vi "Analyze GB.vi"(8 "Integer Tolerance":dbl=0.1, 9 "Twist Angle (Deg)":dbl=60.0, 10 "Grain 2 Orientation":dbl[](array[numeric])=[1.0, 1.0, 1.0], 11 "Grain 1 Orientation":dbl[](array[numeric])=[1.0, 1.0, 1.0]) -> (0 "Misorientation Angle":dbl, 1 "Misorientation Axis, o":dbl[](array[numeric])=[1.0, 1.0, 1.0], 2 "Grain 2 Integers":dbl[](array[numeric])=[1.0, 1.0, 1.0], 3 "Grain 1 Integers":dbl[](array[numeric])=[1.0, 1.0, 1.0], 4 "Tilt Angle (Deg)":dbl, 5 "Suggested Viewing Angle":dbl[](array[numeric])=[1.0, 1.0, 1.0], 6 "Misorientation Matrix":T1, 7 "Viewable?":bool)   [LabVIEW 2010]
uses:
  <vilib>/Analysis/Matrix/Datatypes/RealMatrix.ctl
  <vilib>/Analysis/baseanly.llb/Real A x B.vi
  <vilib>/Analysis/_algsub.llb/Real Matrix Trace.vi
  <vilib>/Analysis/NI_AALPro.lvlib
  <vilib>/Analysis/NI_AALBase.lvlib
  <vilib>/Analysis/Matrix/NI_Matrix.lvlib
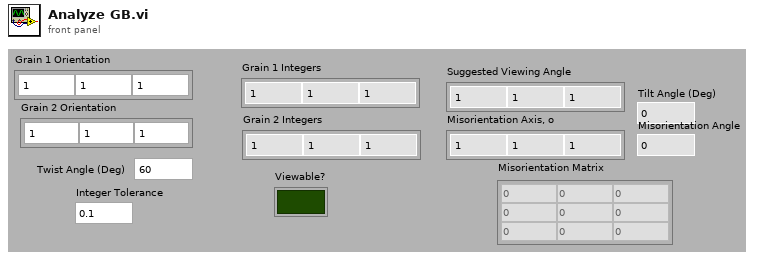
[diagram p1: front panel]
types:
  T1 = typedef "NI_Matrix.lvlib/RealMatrix.ctl" = dbl[][]
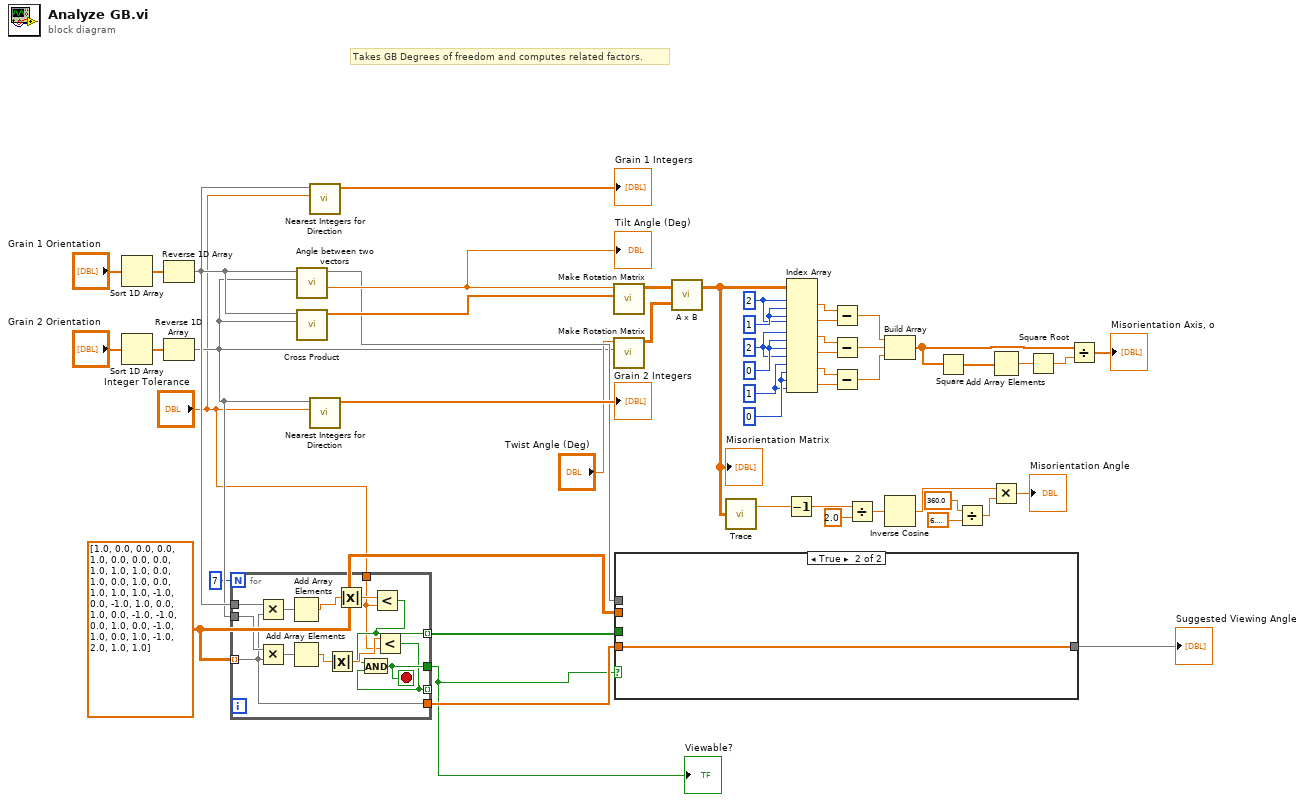
[diagram p0: block diagram]
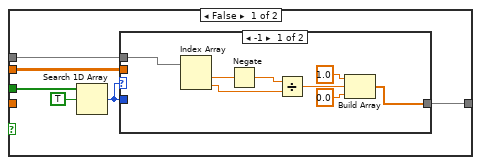
[diagram p2: hidden frame]
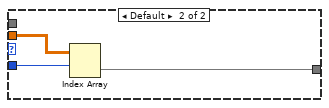
[diagram p3: hidden frame]
diagram:
  w21 = 0 ("index (row)")
  w20 = 1 ("index (row)")
  w23 = 0 ("disabled index (col)")
  w22 = 2 ("index (row)")
  w25 = 1 ("disabled index (col)")
  w24 = 2 ("index (row)")
  w45 = dbl[][] [[1.0, 0.0, 0.0], [0.0, 1.0, 0.0], [0.0, 0.0, 1.0], [1.0, 1.0, 0.0], [1.0, 0.0, 1.0], [0.0, 1.0, 1.0], [1.0, -1.0, 0.0], [-1.0, 1.0, 0.0], [1.0, 0.0, -1.0], [-1.0, 0.0, 1.0], [0.0, -1.0, 1.0], [0.0, 1.0, -1.0], [2.0, 1.0, 1.0]] ("Grain 1 Orientation 2")
  # "Takes GB Degrees of freedom and computes related factors."
  n1 = Sort 1D Array(array="Grain 1 Orientation") -> (sorted array=w48:dbl[])
  n2 = Sort 1D Array(array="Grain 2 Orientation") -> (sorted array=w47:dbl[])
  n3 = Reverse 1D Array(array=w48) -> (reversed array=w13:dbl[])
  n4 = Reverse 1D Array(array=w47) -> (reversed array=w4:dbl[])
  n5 = for {
    N: 7 -> [_]
    tunnel: w13 -> [w62]
    tunnel: w45 -> [w58] mode=indexing
    tunnel: [w58] -> w43
    tunnel: w4 -> [w59]
    tunnel: [w53] -> w46 mode=indexing
    tunnel: [w52] -> _ mode=indexing
    tunnel: [w63] -> w3
    tunnel: "Integer Tolerance" -> [w51]
    stop <- w63 stop-if-true
    n6 = Multiply(x=w62, y=w58) -> (x*y=w61:dbl[])
    n7 = Multiply(x=w59, y=w58) -> (x*y=w60:dbl[])
    n8 = Add Array Elements(numeric array=w61) -> (sum=w57:dbl)
    n9 = Add Array Elements(numeric array=w60) -> (sum=w56:dbl)
    n10 = Absolute Value(x=w56) -> (abs(x)=w54:dbl)
    n11 = Absolute Value(x=w57) -> (abs(x)=w55:dbl)
    n12 = Less?(x=w55, y=w51) -> (x < y?=w53:bool)
    n13 = Less?(x=w54, y=w51) -> (x < y?=w52:bool)
    n14 = And(x=w53, y=w52) -> (x .and. y?=w63:bool)
  }
  "Viewable?" <- w3
  n15 = call "Angle between two vectors.vi"("Vector 2"=w4, "Vector 1"=w13) -> ("Angle (Degrees)"=w30:dbl)  [unwired: 7 in, 2 out]
  "Tilt Angle (Deg)" <- w30
  n16 = call <vilib>:"Cross Product.vi"("B Vector"=w4, "A Vector"=w13) -> ("Cross Product"=w31:dbl[])  [unwired: 8 in, 1 out]
  n17 = call "Nearest Integers for Direction.vi"("Tolerance"="Integer Tolerance", "Direction"=w13) -> ("Nearest Integer Directions"=→"Grain 1 Integers":dbl[])  [unwired: 8 in, 1 out]
  n18 = call "Nearest Integers for Direction.vi"("Tolerance"="Integer Tolerance", "Direction"=w4) -> ("Nearest Integer Directions"=→"Grain 2 Integers":dbl[])  [unwired: 8 in, 1 out]
  n19 = call "Make Rotation Matrix.vi"("Rotation Axis"=w31, "Rotation Angle (Degree)"=w30) -> ("Rotation Matrix"=w32:T1)  [unwired: 9 in]
  n20 = call "Make Rotation Matrix.vi"("Rotation Axis"=w4, "Rotation Angle (Degree)"="Twist Angle (Deg)") -> ("Rotation Matrix"=w42:T1)  [unwired: 9 in]
  n21 = case shown="True" w3 {
    tunnel: [w66 w81] -> w44
    tunnel: w46 -> [w69 _]
    tunnel: w45 -> [w67 _]
    tunnel: w13 -> [w64 _]
    tunnel: w43 -> [_ w81]
    frame False {
      n22 = Search 1D Array(1D array=w69, element=TRUE) -> (index of element=w65:i32)  [unwired: 1 in]
      n23 = case shown="-1" w65 {
        tunnel: w67 -> [_ w80]
        tunnel: w65 -> [_ w79]
        tunnel: [w74 w78] -> w66
        tunnel: w64 -> [w77 _]
        frame -1 {
          n24 = Index Array(array=w77) -> (element #1=w72:dbl, element #2=w73:dbl)  [unwired: 2 in]
          n25 = Negate(x=w72) -> (-x=w71:dbl)
          n26 = Divide(x=w71, y=w73) -> (x/y=w70:dbl)
          n27 = Build Array(1.0 ("element"), w70, 0.0 ("element")) -> (w74:dbl[])
        }
        frame Default {
          n28 = Index Array(array=w80, index (row)=w79) -> (element=w78:dbl[])  [unwired: 1 in]
        }
      }
    }
    frame True {
    }
  }
  "Suggested Viewing Angle" <- w44
  n29 = call-poly <vilib>:"A x B.vi"("B"=w42, "A"=w32) -> ("A x B"=w14:T1)  [unwired: 1 out]
  "Misorientation Matrix" <- w14
  n30 = call-poly <vilib>:"Trace.vi"("Input Matrix"=w14) -> ("trace"=w41:dbl)  [unwired: 1 out]
  n31 = Decrement(x=w41) -> (x-1=w40:dbl)
  n32 = Index Array(array=w14, index (row) #1=w24, index (col) #1=w25, index (row) #2=w25, index (col) #2=w24, index (row) #3=w22, index (col) #3=w23, index (row) #4=w23, index (col) #4=w22, index (row) #5=w20, index (col) #5=w21, index (row) #6=w21, index (col) #6=w20) -> (element #1=w29:dbl, element #2=w28:dbl, element #3=w27:dbl, element #4=w26:dbl, element #5=w19:dbl, element #6=w18:dbl)
  n33 = Subtract(x=w29, y=w28) -> (x-y=w17:dbl)
  n34 = Subtract(x=w27, y=w26) -> (x-y=w16:dbl)
  n35 = Subtract(x=w19, y=w18) -> (x-y=w15:dbl)
  n36 = Divide(x=w40, y=2.0) -> (x/y=w38:dbl)
  n37 = Build Array(w17, w16, w15) -> (w8:dbl[])
  n38 = Inverse Cosine(1:w38) -> (0:w34:dbl)
  n39 = Square(x=w8) -> (x^2=w10:dbl[])
  n40 = Divide(x=360.0, y=6.283185307179586) -> (x/y=w37:dbl)
  n41 = Add Array Elements(numeric array=w10) -> (sum=w11:dbl)
  n42 = Multiply(x=w34, y=w37) -> (x*y=→"Misorientation Angle":dbl)
  n43 = Square Root(x=w11) -> (sqrt(x)=w12:dbl)
  n44 = Divide(x=w8, y=w12) -> (x/y=→"Misorientation Axis, o":dbl[])
